vi "getSerializedData.vi"(0 "reference":refnum<class "ClassNode.lvclass">, 5 "error in (no error)":errorcluster) -> (14 "reference out":refnum<class "ClassNode.lvclass">, 15 "parent":refnum<class "AbstractNode.lvclass">, 16 "children":refnum<class "AbstractNode.lvclass">[](array[class]), 17 "xmlOut":string, 19 "error out":errorcluster)   [LabVIEW 2016, in "ClassNode.lvclass"]
doc: "Gets data to store"
uses:
  <resource>/Framework/Providers/Open_GDS/UML/ClassNode_class/ClassNode.lvclass
  C:/Program Files (x86)/National Instruments/LabVIEW 2016/resource/Framework/Providers/Open_GDS/UML/RectangularNode_class/RectangularNode.lvclass
  C:/Program Files (x86)/National Instruments/LabVIEW 2016/resource/Framework/Providers/Open_GDS/UML/AbstractNode_class/AbstractNode.lvclass
  <resource>/Framework/Providers/Open_GDS/UML/AbstractNode_class/AbstractNode.lvclass
  <resource>/Framework/Providers/Open_GDS/UML/General/Rectangle/Rectangle Rectangle2D.ctl
  <resource>/Framework/Providers/Open_GDS/UML/MultiLineString_class/MultiLineString.lvclass
  <resource>/Framework/Providers/Open_GDS/UML/RectangularNode_class/RectangularNode.lvclass
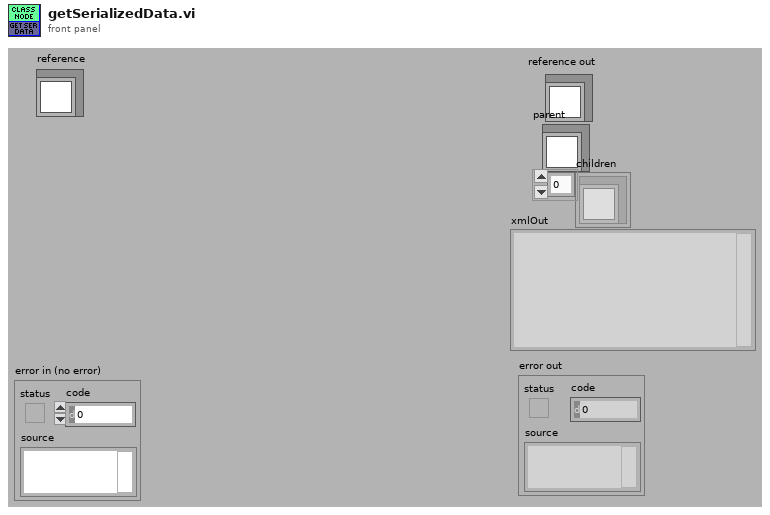
[diagram p1: front panel]
types:
  T1 = typedef "Rectangle Rectangle2D.ctl" = cluster{"x":dbl, "y":dbl, "width":dbl, "height":dbl}
  T2 = cluster{"Base class":cluster{"Base class":cluster{"parent":refnum<k1>, "children":refnum<k1>[], "Hidden":bool}, "bounds":T1}, "midHeight":dbl, "botHeight":dbl, "name":refnum<k1>, "attributes":refnum<k1>, "methods":refnum<k1>, "DEFAULT_COMPARTMENT_HEIGHT":i32, "DEFAULT_WIDTH":i32, "DEFAULT_HEIGHT":i32, "showMethods":bool, "showAttributes":bool, "ClassPath":path}
  T3 = typedef "ClassNode.lvclass/ObjectAttributes.ctl" = cluster{"midHeight":dbl, "botHeight":dbl, "name":refnum<class "MultiLineString.lvclass">, "attributes":refnum<class "MultiLineString.lvclass">, "methods":refnum<class "MultiLineString.lvclass">, "DEFAULT_COMPARTMENT_HEIGHT":i32, "DEFAULT_WIDTH":i32, "DEFAULT_HEIGHT":i32, "showMethods":bool, "showAttributes":bool, "ClassPath":path}
  T4 = typedef "RectangularNode.lvclass/ObjectAttributes.ctl" = cluster{"bounds":T1}
  T5 = typedef "AbstractNode.lvclass/ObjectAttributes.ctl" = cluster{"parent":refnum<class "AbstractNode.lvclass">, "children":refnum<class "AbstractNode.lvclass">[], "Hidden":bool}
  T6 = cluster{"Attributes":cluster{"Base class":cluster{"Base class":cluster{"parent":refnum<k1>, "children":refnum<k1>[], "Hidden":bool}, "bounds":T1}, "midHeight":dbl, "botHeight":dbl, "name":refnum<k1>, "attributes":refnum<k1>, "methods":refnum<k1>, "DEFAULT_COMPARTMENT_HEIGHT":i32, "DEFAULT_WIDTH":i32, "DEFAULT_HEIGHT":i32, "showMethods":bool, "showAttributes":bool, "ClassPath":path}, "text":string, "text":string, "text":string}
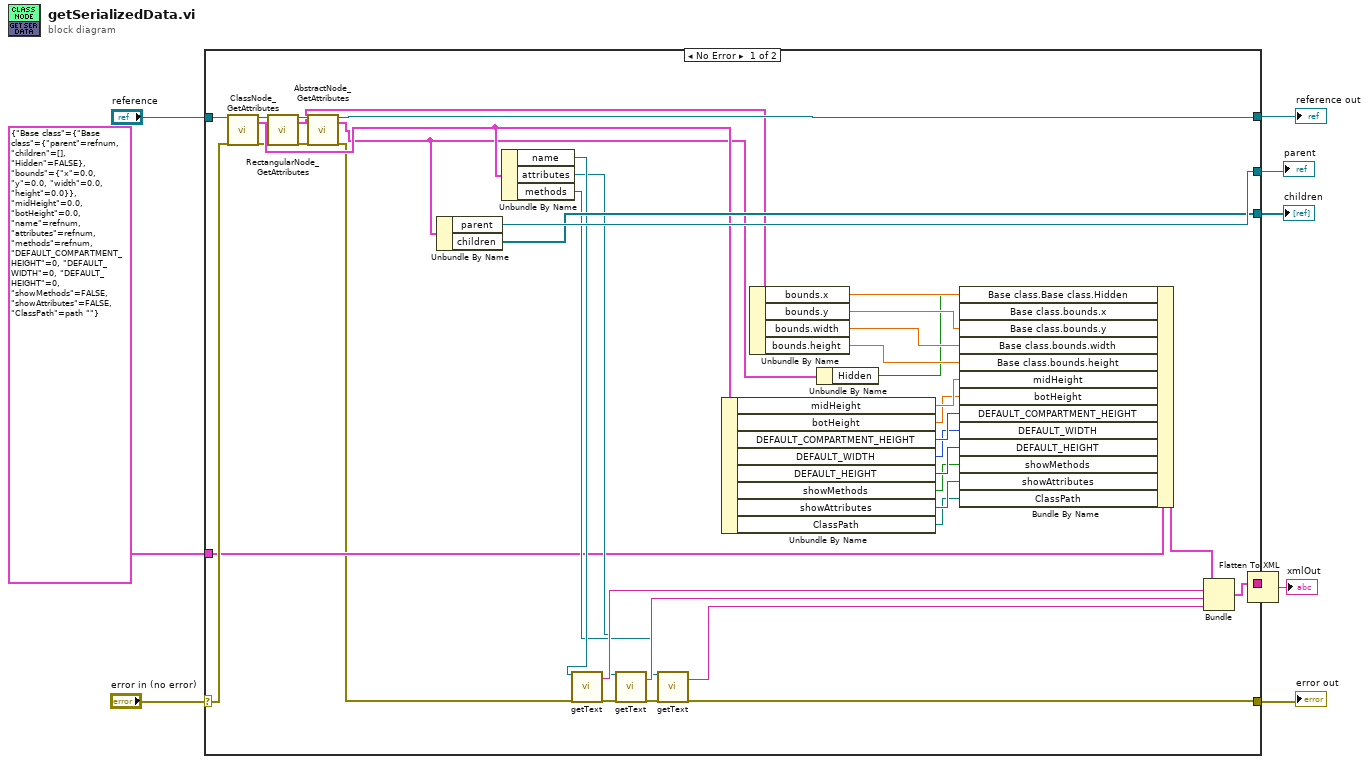
[diagram p0: block diagram]
diagram:
  n1 = case shown="No Error" "error in (no error)" {
    selector: "error in (no error)" -> [w47 w48]
    tunnel: "reference" -> [w46 w49]
    tunnel: [w41 w48] -> w6
    tunnel: [w11 w49] -> w5
    tunnel: [w45 _] -> w4
    tunnel: [w44 _] -> w3
    tunnel: [w43 _] -> w2
    tunnel: T2 {"Base class"={"Base class"={"parent"=refnum, "children"=[], "Hidden"=FALSE}, "bounds"={"x"=0.0, "y"=0.0, "width"=0.0, "height"=0.0}}, "midHeight"=0.0, "botHeight"=0.0, "name"=refnum, "attributes"=refnum, "methods"=refnum, "DEFAULT_COMPARTMENT_HEIGHT"=0, "DEFAULT_WIDTH"=0, "DEFAULT_HEIGHT"=0, "showMethods"=FALSE, "showAttributes"=FALSE, "ClassPath"=path ""} ("Attributes") -> [w32 _]
    frame No Error {
      n2 = call <resource>:"ClassNode_GetAttributes.vi"("reference in"=w46, "error in (no error)"=w47) -> ("reference out"=w16:refnum<class "ClassNode.lvclass">, "Data"=w17:T3, "error out"=w15:errorcluster)  [unwired: 1 in, 14 out]
      n3 = call <resource>:"RectangularNode_GetAttributes.vi"("reference in"=w16, "error in (no error)"=w15) -> ("reference out"=w14:refnum<class "ClassNode.lvclass">, "Data"=w9:T4, "error out"=w13:errorcluster)  [unwired: 14 in, 1 out]
      n4 = call <resource>:"AbstractNode_GetAttributes.vi"("reference in"=w14, "error in (no error)"=w13) -> ("reference out"=w11:refnum<class "ClassNode.lvclass">, "Data"=w10:T5, "error out"=w12:errorcluster)  [unwired: 14 in, 1 out]
      n5 = Unbundle By Name(w10) -> ("parent"=w45:refnum<class "AbstractNode.lvclass">, "children"=w44:refnum<class "AbstractNode.lvclass">[])
      n6 = Unbundle By Name(w17) -> ("name"=w38:refnum<class "MultiLineString.lvclass">, "attributes"=w34:refnum<class "MultiLineString.lvclass">, "methods"=w33:refnum<class "MultiLineString.lvclass">)
      n7 = call-dynamic "getText.vi"("reference"=w38, "error in (no error)"=w12) -> ("text"=w37:string, "error out"=w39:errorcluster)  [unwired: 16 out]
      n8 = call-dynamic "getText.vi"("reference"=w34, "error in (no error)"=w39) -> ("text"=w36:string, "error out"=w40:errorcluster)  [unwired: 16 out]
      n9 = call-dynamic "getText.vi"("reference"=w33, "error in (no error)"=w40) -> ("text"=w35:string, "error out"=w41:errorcluster)  [unwired: 16 out]
      n10 = Unbundle By Name(w17) -> ("midHeight"=w26:dbl, "botHeight"=w25:dbl, "DEFAULT_COMPARTMENT_HEIGHT"=w24:i32, "DEFAULT_WIDTH"=w23:i32, "DEFAULT_HEIGHT"=w22:i32, "showMethods"=w21:bool, "showAttributes"=w20:bool, "ClassPath"=w19:path)
      n11 = Unbundle By Name(w9) -> ("bounds.x"=w30:dbl, "bounds.y"=w29:dbl, "bounds.width"=w28:dbl, "bounds.height"=w27:dbl)
      n12 = Unbundle By Name(w10) -> ("Hidden"=w18:bool)
      n13 = Bundle By Name(cluster=w32, "Base class.Base class.Hidden"=w18, "Base class.bounds.x"=w30, "Base class.bounds.y"=w29, "Base class.bounds.width"=w28, "Base class.bounds.height"=w27, "midHeight"=w26, "botHeight"=w25, "DEFAULT_COMPARTMENT_HEIGHT"=w24, "DEFAULT_WIDTH"=w23, "DEFAULT_HEIGHT"=w22, "showMethods"=w21, "showAttributes"=w20, "ClassPath"=w19) -> (w31:T2)
      n14 = Bundle("Attributes"=w31, "text"=w37, "text"=w36, "text"=w35) -> (w42:T6)  [unwired: 1 out]
      n15 = Flatten To XML(anything=w42) -> (xml string=w43:string)
    }
    frame Error {
    }
  }
  "reference out" <- w5
  "error out" <- w6
  "children" <- w3
  "parent" <- w4
  "xmlOut" <- w2
